vi "Statistic_tail_forming.vi"(1 "Spark/min_IN":dbl[](array[numeric])) -> (0 "Spark/min_OUT":dbl[](array[numeric]))   [LabVIEW 2018]
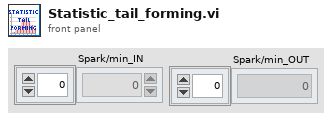
[diagram p1: front panel]
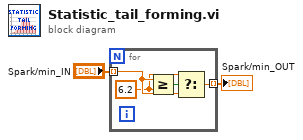
[diagram p0: block diagram]
diagram:
  n1 = for {
    tunnel: "Spark/min_IN" -> [w4] mode=indexing
    tunnel: [w5] -> w1 mode=indexing
    w3 = 6.2 ("y")
    n2 = Greater Or Equal?(x=w4, y=w3) -> (x >= y?=w6:bool)
    n3 = Select(t=w3, s=w6, f=w4) -> (s? t:f=w5:dbl)
  }
  "Spark/min_OUT" <- w1
